vi "Autonomous.vi"   [LabVIEW 2019]
doc: "This VI starts when autonomous period begins, and will automatically be terminated when it ends. You can carry out timed or sensor driven operations directly to I/O or to subsystems without needing to return to the caller."
uses:
  <vilib>/Rock Robotics/Network Tables/NT Read String.vi
  <vilib>/Rock Robotics/Network Tables/NT Read Number.vi
  Framework/Robot Global Data.vi
types:
  T1 = typedef "Command Status Info.ctl" = cluster{"Name":string, "Status":T2, "notifier out":T3}
  T2 = typedef "Completion Status.ctl" = enum16{"Successful", "Aborted", "Incomplete"}
  T3 = typedef "Completion Notifier.ctl" = refnum<notifier>
  T4 = typedef "WPI_JoystickDevRef.ctl" = cluster{"Device":T5}
  T5 = typedef "WPI_JoystickDeviceEnum.ctl" = enum16{"USB 0", "USB 1", "USB 2", "USB 3", "USB 4", "USB 5"}
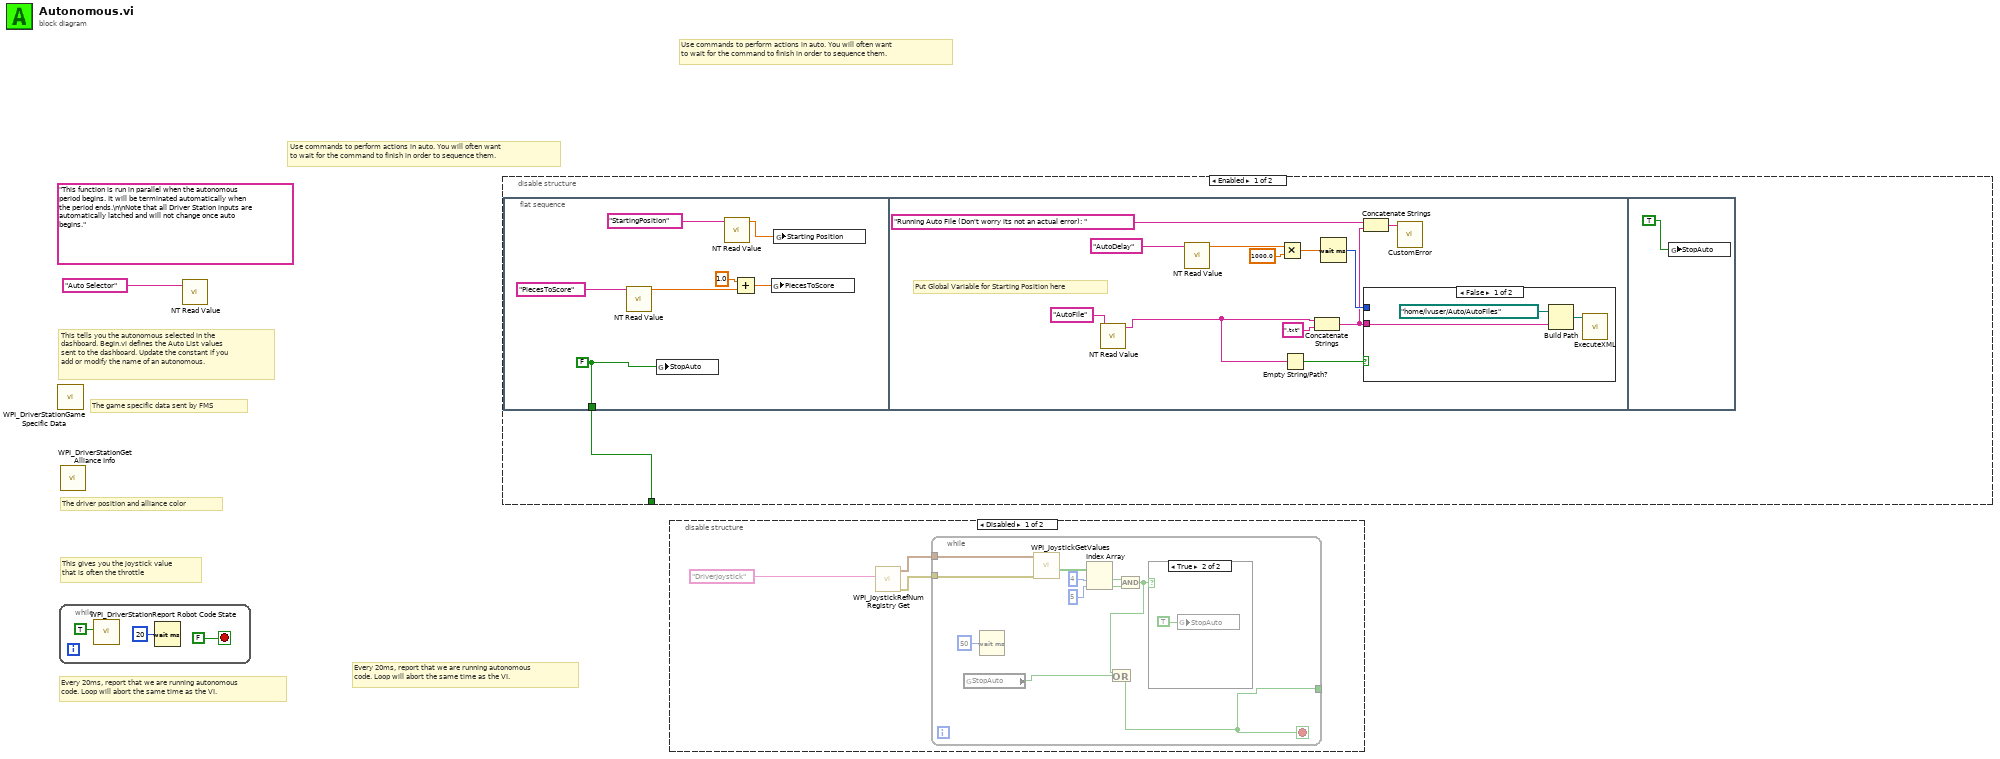
[diagram p0: block diagram]
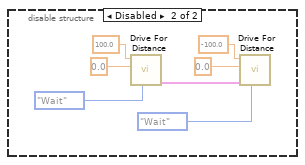
[diagram p5: hidden frame]
diagram:
  (unwired) "This function is run in parallel when the autonomous period begins. It will be terminated automatically when the period ends.\n\nNote that all Driver Station inputs are automatically latched and will not change once auto begins."
  # "Every 20ms, report that we are running autonomous\ncode. Loop will abort the same time as the VI."
  # "Use commands to perform actions in auto. You will often want\nto wait for the command to finish in order to sequence them."
  # "The game specific data sent by FMS"
  # "This tells you the autonomous selected in the \ndashboard. Begin.vi defines the Auto List values\nsent to the dashboard. Update the constant if you\nadd or modify the name of an autonomous."
  # "Every 20ms, report that we are running autonomous\ncode. Loop will abort the same time as the VI."
  # "This gives you the joystick value\nthat is often the throttle"
  # "Use commands to perform actions in auto. You will often want\nto wait for the command to finish in order to sequence them."
  # "The driver position and alliance color"
  n1 = call <vilib>:"WPI_DriverStationGame Specific Data.vi"() -> ()  [unwired: 11 in, 1 out]
  n2 = while {
    stop <- FALSE stop-if-true
    n3 = call <vilib>:"WPI_DriverStationReport Robot Code State.vi"("Autonomous"=TRUE) -> ()  [unwired: 10 in, 1 out]
    n4 = Wait (ms)(milliseconds to wait=u32 20) -> ()  [unwired: 1 out]
  }
  n5 = call <vilib>:"WPI_DriverStationGet Alliance Info.vi"() -> ()  [unwired: 12 out]
  n6 = call-poly <vilib>:"NT Read Value.vi"("Name"="Auto Selector") -> ()  [unwired: 9 in, 2 out]
  n7 = disable-structure shown="Enabled" {
    disable-tunnel: [w5 _] -> _
    frame Enabled {
      n8 = flat-sequence {
        tunnel: [w8] -> w5
        frame #0 {
          w8 = FALSE
          n9 = call-poly <vilib>:"NT Read Value.vi"("Name"="PiecesToScore") -> ("Numeric"=w9:dbl)  [unwired: 9 in, 1 out]
          n10 = global write "Robot Global Data.vi" "StopAuto"(w8) -> ()
          n11 = call-poly <vilib>:"NT Read Value.vi"("Name"="StartingPosition") -> ("Numeric"=w6:dbl)  [unwired: 9 in, 1 out]
          n12 = Add(x=1.0, y=w9) -> (x+y=w7:dbl)
          n13 = global write "Robot Global Data.vi" "PiecesToScore"(w7) -> ()
          n14 = global write "Robot Global Data.vi" "Starting Position"(w6) -> ()
        }
        frame #1 {
          # "Put Global Variable for Starting Position here"
          n15 = call-poly <vilib>:"NT Read Value.vi"("Name"="AutoFile") -> ("String"=w13:string)  [unwired: 9 in, 1 out]
          n16 = call-poly <vilib>:"NT Read Value.vi"("Name"="AutoDelay") -> ("Numeric"=w16:dbl)  [unwired: 9 in, 1 out]
          n17 = Multiply(x=w16, y=1000.0) -> (x*y=w15:dbl)
          n18 = Empty String/Path?(string/path=w13) -> (empty?=w24:bool)
          n19 = Concatenate Strings(w13, ".txt" ("string")) -> (w19:string)
          n20 = Wait (ms)(milliseconds to wait=w15) -> (millisecond timer value=w23:u32)
          n21 = Concatenate Strings("Running Auto File (Don't worry its not an actual error): " ("string"), w19) -> (w22:string)
          n22 = case shown="False" w24 {
            tunnel: w19 -> [w25 _]
            tunnel: w23 -> [_ _]
            frame False {
              n23 = Build Path(base path=path "/home/lvuser/Auto/AutoFiles", name or relative path=w25) -> (appended path=w27:path)
              n24 = call "ExecuteXML.vi"("Auto File Path"=w27) -> ()  [unwired: 10 in, 1 out]
            }
            frame True {
            }
          }
          n25 = call "CustomError.vi"("String"=w22) -> ()  [unwired: 10 in, 1 out]
        }
        frame #2 {
          n26 = global write "Robot Global Data.vi" "StopAuto"(TRUE) -> ()
        }
      }
    }
    frame Disabled {
      n27 = call "Drive For Distance.vi"("Synchronication"=enum16{"Start", "Wait"}."Wait", 10:0.0 ("Angle"), "Distance"=100.0) -> ("Command Info Out"=w29:T1)  [unwired: 8 in]
      n28 = call "Drive For Distance.vi"("Synchronication"=enum16{"Start", "Wait"}."Wait", "Command Info In"=w29, 10:0.0 ("Angle"), "Distance"=-100.0) -> ()  [unwired: 7 in, 1 out]
    }
  }
  n29 = disable-structure shown="Disabled" {
    frame Disabled {
      n30 = call <vilib>:"WPI_JoystickRefNum Registry Get.vi"("refnum name"="DriverJoystick") -> ("error out"=w37:errorcluster, "JoystickDevRef"=w38:T4)  [unwired: 9 in]
      n31 = while {
        tunnel: w37 -> [w44]
        tunnel: w38 -> [w43]
        tunnel: [w40] -> _
        stop <- w40 stop-if-true
        n32 = global read "Robot Global Data.vi" "StopAuto"() -> (w39:bool)
        n33 = Wait (ms)(milliseconds to wait=u32 50) -> ()  [unwired: 1 out]
        n34 = call <vilib>:"WPI_JoystickGetValues.vi"("error in (no error)"=w44, "JoystickDevRef"=w43) -> ("Buttons"=w47:bool[])  [unwired: 5 in, 4 out]
        n35 = Index Array(array=w47, index #1=4 ("index"), index #2=5 ("index")) -> (element #1=w48:bool, element #2=w49:bool)
        n36 = And(x=w48, y=w49) -> (x .and. y?=w41:bool)
        n37 = Or(x=w41, y=w39) -> (x .or. y?=w40:bool)
        n38 = case shown="True" w41 {
          frame False {
          }
          frame True {
            n39 = global write "Robot Global Data.vi" "StopAuto"(TRUE ("StopAuto")) -> ()
          }
        }
      }
    }
    frame Enabled {
    }
  }
